vi "fgv_measure_contR.vi"(7 "cmd":T2, 8 "error in (no error)":errorcluster, 11 "measure_ContR In":T1) -> (0 "error out":errorcluster, 3 "measure_ContR Out":T1)   [LabVIEW 2019]
uses:
  _ctrl/rw.ctl
  data_contR.ctl
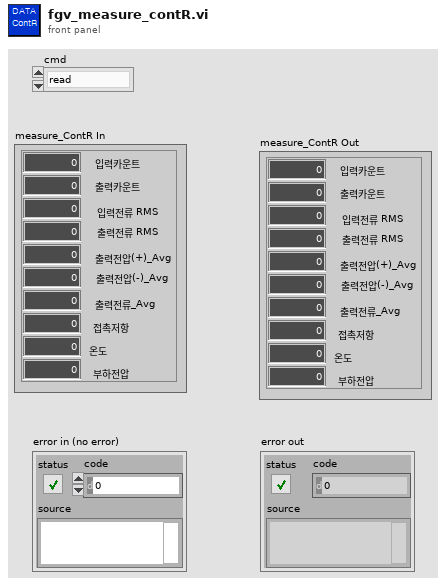
[diagram p1: front panel]
types:
  T1 = typedef "data_contR.ctl" = cluster{"입력카운트":dbl, "출력카운트":dbl, "입력전류 RMS":dbl, "출력전류 RMS":dbl, "출력전압(+)_Avg":dbl, "출력전압(-)_Avg":dbl, "출력전류_Avg":dbl, "접촉저항":dbl, "온도":dbl, "부하전압":dbl}
  T2 = typedef "rw.ctl" = enum16{"read", "write"}
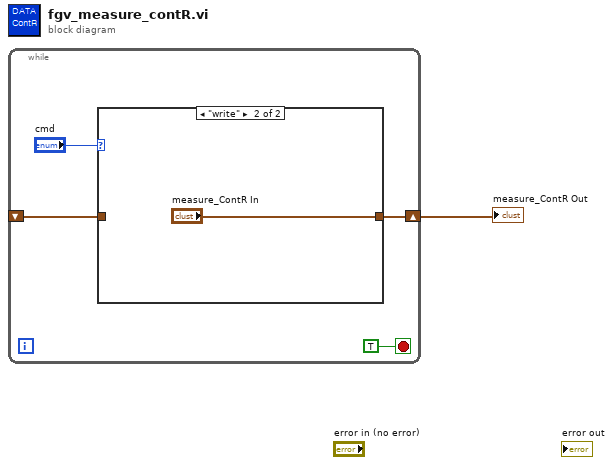
[diagram p0: block diagram]
diagram:
  n1 = while {
    shift-right: [w3] -> w1
    shift-left: _ -> [w2]
    stop <- TRUE stop-if-true
    n2 = case shown="\"write\"" "cmd" {
      tunnel: [w6 "measure_ContR In"] -> w3
      tunnel: w2 -> [w6 _]
      frame "read", Default {
      }
      frame "write" {
      }
    }
  }
  "measure_ContR Out" <- w1
